vi "LVClass_CameraSet Get Parameter Option.vi"(0 "CameraSet.lvclass":refnum<class "CameraSet.lvclass">, 5 "parameter_name":string, 11 "error in (no error)":errorcluster) -> (1 "Settable-Gettable?":cluster{"Settable":bool, "Gettable":bool}, 3 "Settable-Gettable on fly?":cluster{"Settable":bool, "Gettable":bool}, 4 "CameraSet.lvclass":refnum<class "CameraSet.lvclass">, 6 "is_connection_parameter?":bool, 12 "String enum":bool, 13 "DefaultValueExist":bool, 14 "minmax":bool, 15 "error out":errorcluster)   [LabVIEW 2020, in "CameraSet.lvclass"]
doc: "Camera parameter options getter given its name which should have been read\nwith Imop_CameraSet_GetParameterName.\n\n--------------------------------------------------------------------------------\n\n<B>camera_setIn </B> : CameraSet object.\n<B>camera_setOut </B> : CameraSet object.\n<B>parameter_name </B> : Parameter name.\n<B>is_settable </B> : Parameter value is writeable.\n<B>is_gettable </B> : Parameter value is readable.\n<B>has_default_value </B> : Parameter has a default value.\n<B>has_limits </B> : If parameter is a number, its value is to be selected between a min and a max\n value.\n<B>is_string_enum </B> : If parameter is a string, its value is to be selected in a finite set of\n values.\n<B>is_settable_on_fly </B> : Parameter is writeable while camera is running, and a value change is taken\n into account asap.\n<B>is_gettable_on_fly </B> : Parameter is readable while camera is running, and the return value will be\n the one currently used.\n<B>ErrorIn </B> : Error\n<B>ErrorOut </B> : Error\n\n--------------------------------------------------------------------------------"
uses:
  CameraSet.lvclass
  CameraSet.lvclass/CameraSet.ctl
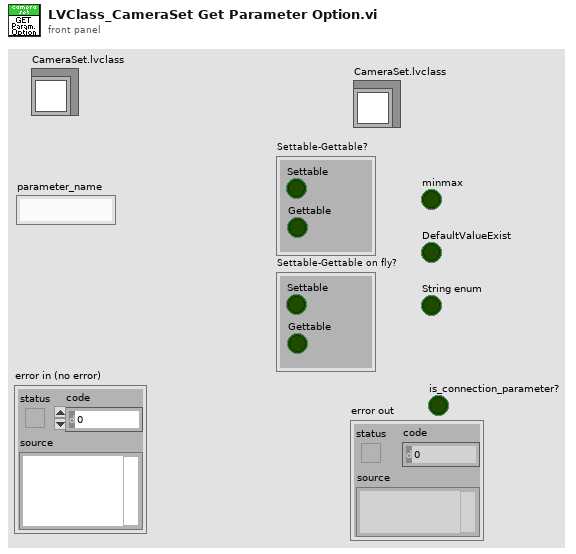
[diagram p1: front panel]
types:
  T1 = typedef "ClassID.ctl" = i64
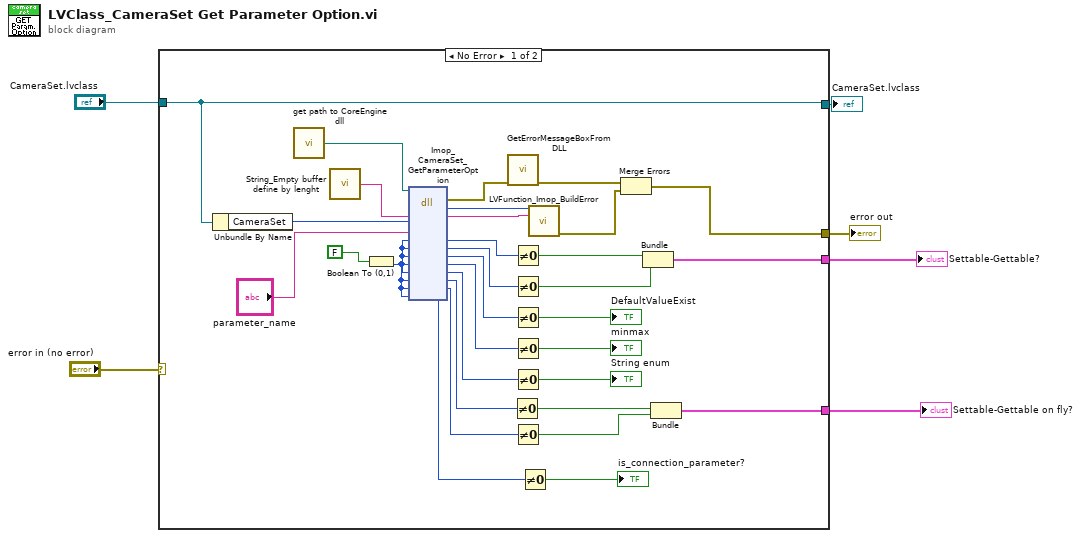
[diagram p0: block diagram]
diagram:
  n1 = case shown="No Error" "error in (no error)" {
    selector: "error in (no error)" -> [_ w38]
    tunnel: "CameraSet.lvclass" -> [w22 w39]
    tunnel: [w22 w39] -> w4
    tunnel: [w18 w38] -> w3
    tunnel: [w16 _] -> w2
    tunnel: [w10 _] -> w1
    frame No Error {
      n2 = Unbundle By Name(w22) -> ("CameraSet"=w21:T1)
      n3 = call "get path to CoreEngine dll.vi"() -> ("path to c_interface_vc100.dll"=w33:path)  [unwired: 12 in, 3 out]
      n4 = call "String_Empty buffer define by lenght.vi"() -> ("Empty buffer"=w35:string)  [unwired: 1 in]
      n5 = Boolean To (0,1)(Boolean=FALSE) -> (0, 1=w7:i16)
      n6 = dll-call lib="D:/2_trunk/temp_core_engine/DLLs/ImopEngine4_vc100.dll" fn="Imop_CameraSet_GetParameterOption"(path in=w33, "message"=w35, "objet"=w21, "parameter_name"="parameter_name", "Settable"=w7, "Gettable"=w7, "DefaultValueExist"=w7, "minmax"=w7, "StringEnum"=w7, "Settable_onfly"=w7, "Gettable_onfly"=w7, "ConnectionParameter"=w7) -> (error out=w32:errorcluster, "return type"=w37:i32, "message"=w36:string, "Settable"=w30:u8, "Gettable"=w29:u8, "DefaultValueExist"=w28:u8, "minmax"=w26:u8, "StringEnum"=w24:u8, "Settable_onfly"=w14:u8, "Gettable_onfly"=w13:u8, "ConnectionParameter"=w8:u8)  [unwired: 4 in, 1 out]
      n7 = call "GetErrorMessageBoxFromDLL.vi"("error IN"=w32) -> ("error OUT"=w20:errorcluster)  [unwired: 10 in]
      n8 = Not Equal To 0?(x=w14) -> (x != 0?=w12:bool)
      n9 = Not Equal To 0?(x=w30) -> (x != 0?=w17:bool)
      n10 = Not Equal To 0?(x=w29) -> (x != 0?=w15:bool)
      n11 = Not Equal To 0?(x=w28) -> (x != 0?=→"DefaultValueExist":bool)
      n12 = Not Equal To 0?(x=w26) -> (x != 0?=→"minmax":bool)
      n13 = Not Equal To 0?(x=w24) -> (x != 0?=→"String enum":bool)
      n14 = Not Equal To 0?(x=w13) -> (x != 0?=w11:bool)
      n15 = Not Equal To 0?(x=w8) -> (x != 0?=→"is_connection_parameter?":bool)
      n16 = call "LVFunction_Imop_BuildError.vi"("code"=w37, "String to Prepend to source (\"\")"=w36) -> ("error out"=w19:errorcluster)  [unwired: 13 in]
      n17 = Merge Errors(w20, w19) -> (w18:errorcluster)
      n18 = Bundle(w17, w15) -> (w16:cluster{bool, bool})  [unwired: 1 in]
      n19 = Bundle(w12, w11) -> (w10:cluster{bool, bool})  [unwired: 1 in]
    }
    frame Error {
    }
  }
  "CameraSet.lvclass" <- w4
  "error out" <- w3
  "Settable-Gettable?" <- w2
  "Settable-Gettable on fly?" <- w1
